vi "CSM Execute - Rescan CSM-VI.vi"(6 "Mouse Position":T1, 8 "User VI Ref":refnum<vi>, 9 "Menu Item Tag Suffix":string, 10 "Remaining Items":refnum<vi>[](array[refnum]), 11 "Affected Items":T2) -> (0 "Fail transaction?":bool)   [LabVIEW 2017]
doc: "This VI is part of a plug-in for modifying the LabVIEW shortcut menus. This is the execute VI which is called when the shortcut menu is chosen by the user. It performs the action of the selected menu item."
uses:
  CSM Execute - Shortcut Menu Plug-In.ctl
  <vilib>/Utility/miscctls.llb/LVPositionTypeDef.ctl
panel:
  # "All controls on this panel except \"Affected Items\" have been locked to prevent accidental edits. Changing the control names or types, other than the elements of the \"Affected Items\" cluster will make the VI unusable as a menu plugin.\n\nSee Context Help for each control for details about its use."
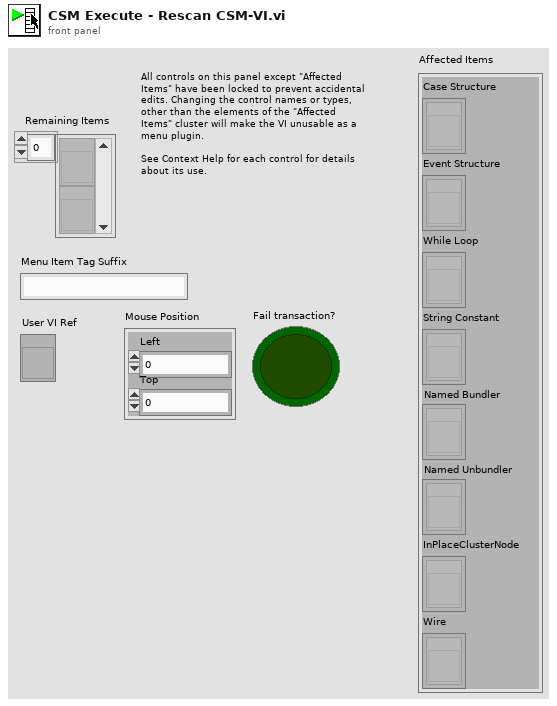
[diagram p1: front panel]
types:
  T1 = typedef "LVPositionTypeDef.ctl" = cluster{"Left":i32, "Top":i32}
  T2 = typedef "CSM Execute - Shortcut Menu Plug-In.ctl" = cluster{"Case Structure":refnum<vi>[], "Event Structure":refnum<vi>[], "While Loop":refnum<vi>[], "String Constant":refnum<vi>[], "Named Bundler":refnum<vi>[], "Named Unbundler":refnum<vi>[], "InPlaceClusterNode":refnum<vi>[], "Wire":refnum<vi>[]}
  T3 = typedef "LVRectTypeDef.ctl" = cluster{"Left":i16, "Top":i16, "Right":i16, "Bottom":i16}
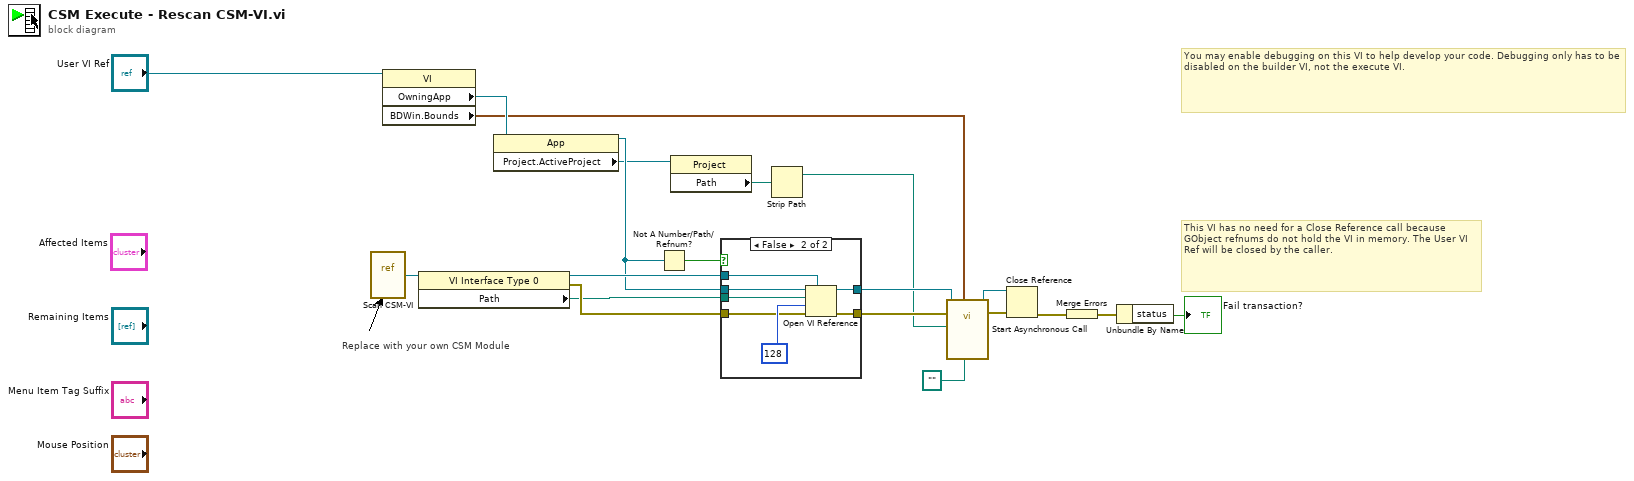
[diagram p0: block diagram]
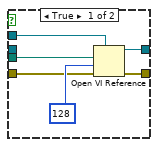
[diagram p2: hidden frame]
diagram:
  # "Replace with your own CSM Module"
  # "You may enable debugging on this VI to help develop your code. Debugging only has to be disabled on the builder VI, not the execute VI."
  # "This VI has no need for a Close Reference call because GObject refnums do not hold the VI in memory. The User VI Ref will be closed by the caller."
  n1 = vi-ref "Scan CSM-VI.vi"() -> (w12:refnum<vi>)
  n2 = property class="VI"(reference="User VI Ref") -> ("OwningApp"=w7:refnum<vi>, "BDWin.Bounds"=w6:T3)  [unwired: 1 in, 2 out]
  n3 = property class="VI Interface Type 0"(reference=w12) -> (reference out=w16:refnum<vi>, error out=w14:errorcluster, "Path"=w13:path)  [unwired: 1 in]
  n4 = property class="App"(reference=w7) -> (reference out=w5:refnum<vi>, "Project.ActiveProject"=w4:refnum<vi>)  [unwired: 1 in, 1 out]
  n5 = Not A Number/Path/Refnum?(number/path/refnum=w5) -> (NaN/Path/Refnum?=w8:bool)
  n6 = property class="Project"(reference=w4) -> ("Path"=w3:path)  [unwired: 1 in, 2 out]
  n7 = case shown="False" w8 {
    tunnel: w16 -> [w25 w32]
    tunnel: [w24 w31] -> w15
    tunnel: w14 -> [w23 w30]
    tunnel: w13 -> [w22 w29]
    tunnel: [w21 w28] -> w11
    tunnel: w5 -> [_ w27]
    frame True {
      n8 = Open VI Reference(type specifier VI Refnum (for type only)=w25, vi path=w22, options=128, error in (no error)=w23) -> (vi reference=w24:refnum<vi>, error out=w21:errorcluster)  [unwired: 2 in]
    }
    frame False {
      n9 = Open VI Reference(type specifier VI Refnum (for type only)=w32, application reference (local)=w27, vi path=w29, options=128, error in (no error)=w30) -> (vi reference=w31:refnum<vi>, error out=w28:errorcluster)  [unwired: 1 in]
    }
  }
  n10 = Strip Path(path=w3) -> (stripped path=w2:path)  [unwired: 1 out]
  n11 = call-by-ref "Start Asynchronous Call"(reference=w15, error in=w11, "Config Path"=path "", "Block Diagram Window:Window Bounds"=w6, "root"=w2) -> (reference out=w18:refnum<vi>, error out=w17:errorcluster)  [unwired: 8 in, 1 out]
  n12 = Close Reference(reference=w18, error in (no error)=w17) -> (error out=w10:errorcluster)
  n13 = Merge Errors(w10) -> (w19:errorcluster)
  n14 = Unbundle By Name(w19) -> ("status"=→"Fail transaction?":bool)
